vi "Mock Circulation Loop.vi"() -> ()   [LabVIEW 2024]
uses:
  <vilib>/DAQmx/write.llb/DAQmx Write (Analog DBL 1Chan 1Samp).vi
  <vilib>/DAQmx/read.llb/DAQmx Read (Analog 1D DBL NChan 1Samp).vi
  <vilib>/DAQmx/write.llb/DAQmx Write (Digital 1D Bool NChan 1Samp 1Line).vi
  <vilib>/DAQmx/create/channels.llb/DAQmx Create Channel (DO-Digital Output).vi
  <vilib>/DAQmx/miscellaneous.llb/DAQmx Fill In Error Info.vi
  <vilib>/DAQmx/create/channels.llb/DAQmx Create Channel (AI-Voltage-Basic).vi
  <vilib>/DAQmx/create/channels.llb/DAQmx Create Channel (AO-Voltage-Basic).vi
  <vilib>/Utility/file.llb/Write Delimited Spreadsheet (string).vi
  <vilib>/Utility/file.llb/Write Delimited Spreadsheet (DBL).vi
panel:
  in  "Set pressure Hybrid Heart (Bar)":dbl
  in  "Analog output pressure regulator":tag
  out "Actual pressure to Hybrid Heart (Bar)":dbl
  out "Flow sensors":cluster{dbl[], dbl[]}[](graph)
  in  "Seconds per data point":dbl
  out "Pressure sensors":cluster{dbl[], dbl[]}[](graph)
  out "Elapsed time":dbl
  in  "Input port all sensors":tag
  in  "Start/Stop solenoid valves":bool
  in  "Closed time (ms)":dbl
  in  "Open time (ms)":dbl
  in  "STOP":bool
  in  "line grouping":i32(ring)=1 items=["one channel for each line", "one channel for all lines"]
  in  "Port input Solenoid valve":tag
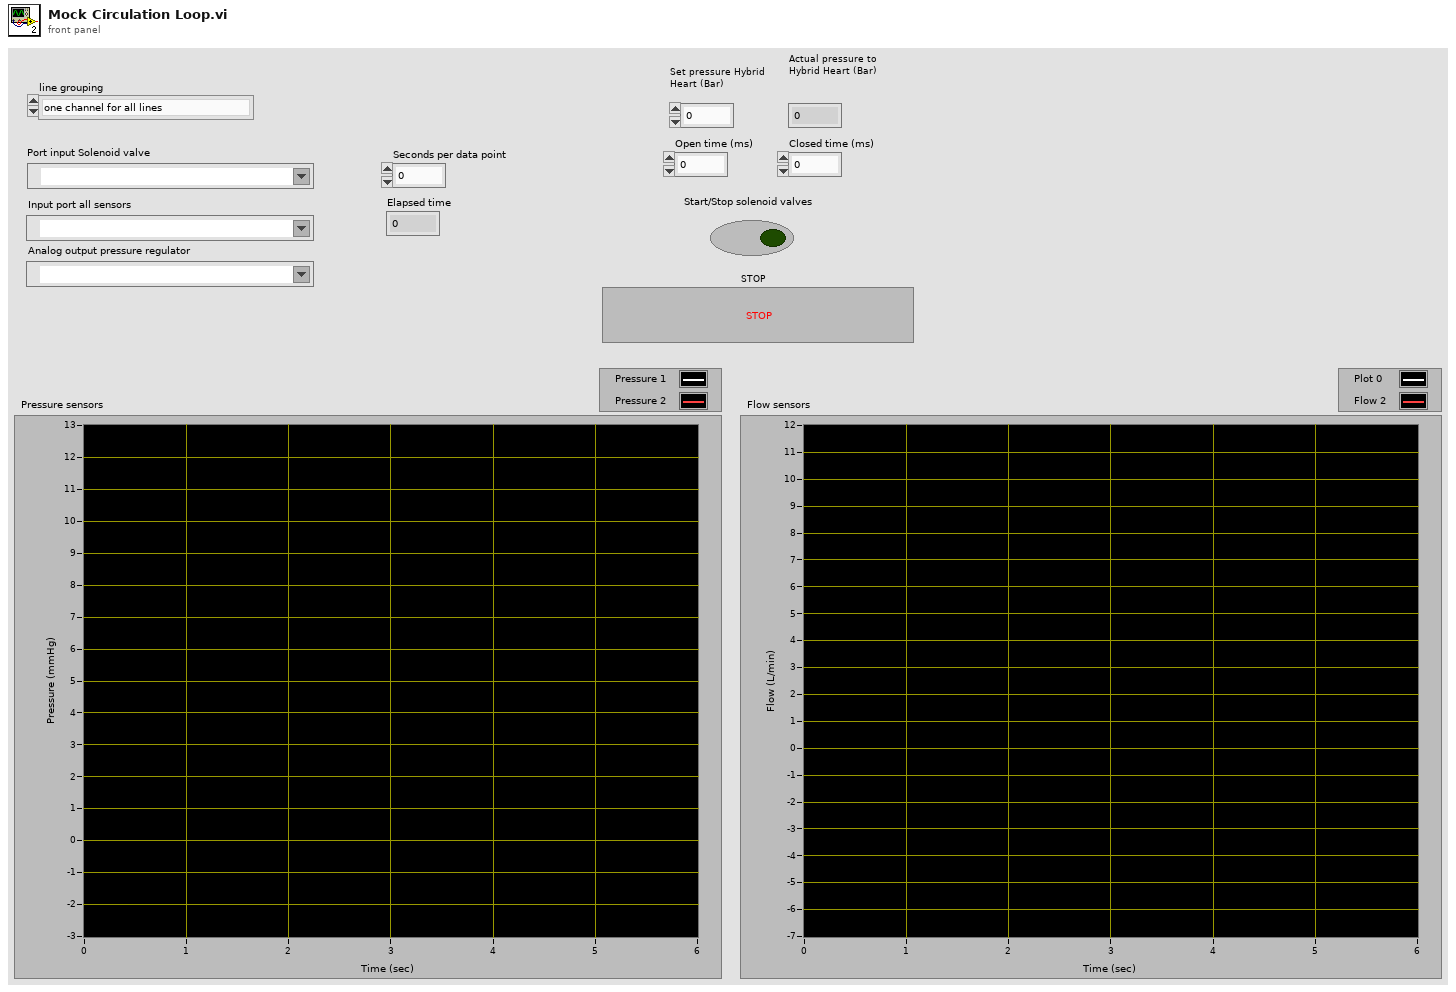
[diagram p1: front panel]
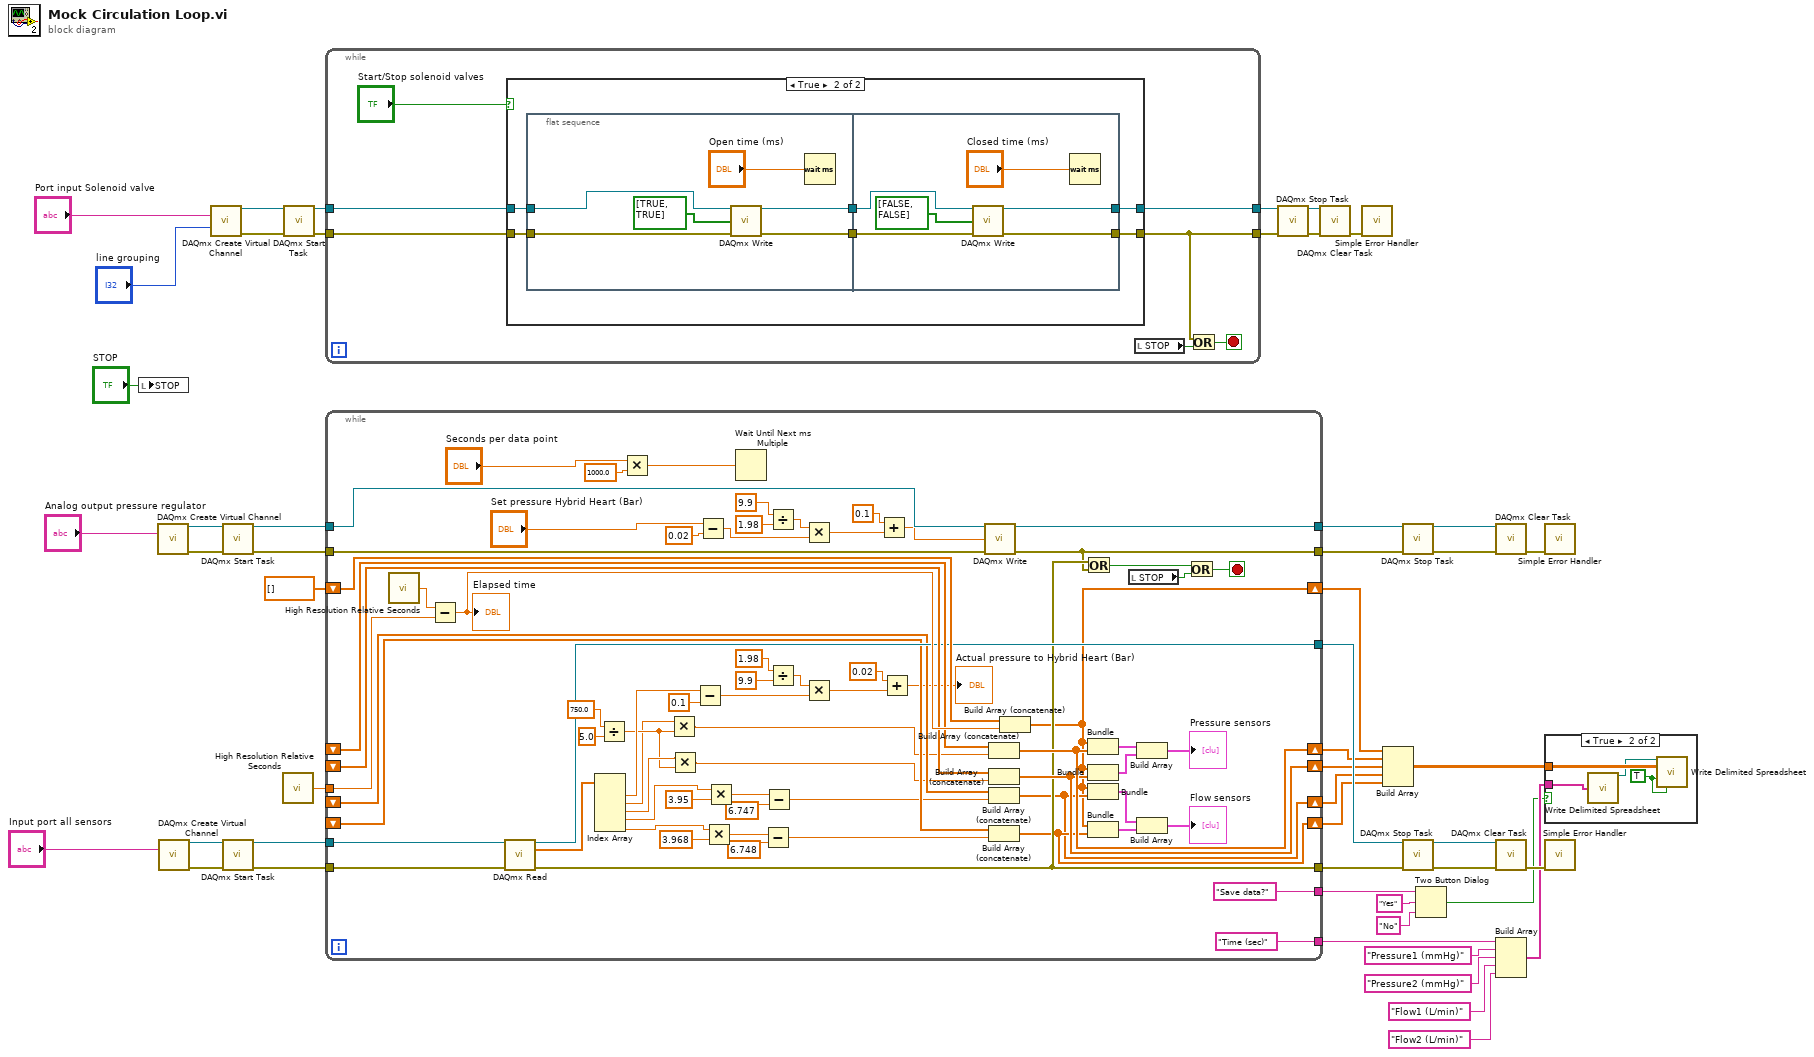
[diagram p0: block diagram]
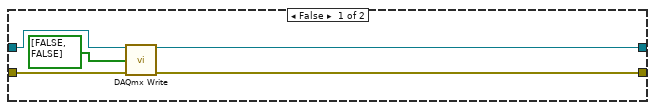
[diagram p3: hidden frame]
diagram:
  n1 = local write "STOP"("STOP") -> ()
  n2 = call-poly <vilib>:"DAQmx Create Virtual Channel.vi"("physical channels"="Analog output pressure regulator") -> ("task out"=w27:refnum<k21>, "error out"=w26:errorcluster)  [unwired: 13 in]
  n3 = call-poly <vilib>:"DAQmx Create Virtual Channel.vi"("physical channels"="Input port all sensors") -> ("task out"=w36:refnum<k21>, "error out"=w35:errorcluster)  [unwired: 13 in]
  n4 = call-poly <vilib>:"DAQmx Create Virtual Channel.vi"("lines"="Port input Solenoid valve", "line grouping"="line grouping") -> ("task out"=w48:refnum<k21>, "error out"=w49:errorcluster)  [unwired: 12 in]
  n5 = call <vilib>:"DAQmx Start Task.vi"("task/channels in"=w27, "error in"=w26) -> ("task out"=w23:refnum<k21>, "error out"=w24:errorcluster)  [unwired: 12 in]
  n6 = call <vilib>:"DAQmx Start Task.vi"("task/channels in"=w36, "error in"=w35) -> ("task out"=w34:refnum<k21>, "error out"=w33:errorcluster)  [unwired: 12 in]
  n7 = call <vilib>:"High Resolution Relative Seconds.vi"() -> ("relative seconds"=w38:dbl)
  n8 = call <vilib>:"DAQmx Start Task.vi"("task/channels in"=w48, "error in"=w49) -> ("task out"=w46:refnum<k21>, "error out"=w45:errorcluster)  [unwired: 12 in]
  n9 = while {
    tunnel: w46 -> [w56]
    tunnel: w45 -> [w55]
    tunnel: [w52] -> w43
    tunnel: [w54] -> w42
    stop <- w53 stop-if-true
    n10 = case shown="True" "Start/Stop solenoid valves" {
      tunnel: w56 -> [w62 w66]
      tunnel: w55 -> [w61 w65]
      tunnel: [w59 w64] -> w52
      tunnel: [w58 w63] -> w54
      frame False {
        n11 = call-poly <vilib>:"DAQmx Write.vi"("task/channels in"=w62, "data"=bool[] [FALSE, FALSE], "error in"=w61) -> ("task out"=w58:refnum<k21>, "error out"=w59:errorcluster)  [unwired: 10 in, 1 out]
      }
      frame True {
        n12 = flat-sequence {
          tunnel: w66 -> [w74]
          tunnel: w65 -> [w73]
          tunnel: [w71] -> w68
          tunnel: [w70] -> w67
          tunnel: w68 -> [w79]
          tunnel: w67 -> [w78]
          tunnel: [w77] -> w63
          tunnel: [w76] -> w64
          frame #0 {
            n13 = call-poly <vilib>:"DAQmx Write.vi"("task/channels in"=w74, "data"=bool[] [TRUE, TRUE], "error in"=w73) -> ("task out"=w71:refnum<k21>, "error out"=w70:errorcluster)  [unwired: 10 in, 1 out]
            n14 = Wait (ms)(milliseconds to wait="Open time (ms)") -> ()  [unwired: 1 out]
          }
          frame #1 {
            n15 = call-poly <vilib>:"DAQmx Write.vi"("task/channels in"=w79, "data"=bool[] [FALSE, FALSE], "error in"=w78) -> ("task out"=w77:refnum<k21>, "error out"=w76:errorcluster)  [unwired: 10 in, 1 out]
            n16 = Wait (ms)(milliseconds to wait="Closed time (ms)") -> ()  [unwired: 1 out]
          }
        }
      }
    }
    n17 = local read "STOP"() -> (w51:bool)
    n18 = Or(x=w52, y=w51) -> (x .or. y?=w53:bool)
  }
  n19 = while {
    tunnel: w34 -> [w151]
    tunnel: w33 -> [w150]
    tunnel: w38 -> [w145]
    shift-right: [w128] -> w17
    shift-left: dbl[] [] -> [w143]
    shift-right: [w139] -> w16
    shift-left: _ -> [w141]
    shift-right: [w138] -> w15
    shift-left: _ -> [w140]
    tunnel: [w134] -> w32
    tunnel: [w133] -> w31
    shift-right: [w129] -> w14
    shift-left: _ -> [w132]
    shift-right: [w130] -> w13
    shift-left: _ -> [w131]
    tunnel: w24 -> [w124]
    tunnel: w23 -> [w123]
    tunnel: [w121] -> w19
    tunnel: [w122] -> w18
    tunnel: ["Time (sec)"] -> w6
    tunnel: ["Save data?" ("message")] -> w2
    stop <- w100 stop-if-true
    n20 = call <vilib>:"High Resolution Relative Seconds.vi"() -> ("relative seconds"=w146:dbl)
    n21 = Subtract(x=w146, y=w145) -> (x-y=w144:dbl)
    "Elapsed time" <- w144
    n22 = call-poly <vilib>:"DAQmx Read.vi"("task/channels in"=w151, "error in"=w150) -> ("task out"=w134:refnum<k21>, "data"=w142:dbl[], "error out"=w133:errorcluster)  [unwired: 11 in]
    n23 = Index Array(array=w142) -> (element #1=w120:dbl, element #2=w81:dbl, element #3=w87:dbl, element #4=w83:dbl, element #5=w82:dbl)  [unwired: 5 in]
    n24 = Divide(x=750.0, y=5.0) -> (x/y=w84:dbl)
    n25 = Multiply(x="Seconds per data point", y=1000.0) -> (x*y=w149:dbl)
    n26 = Multiply(x=w81, y=w84) -> (x*y=w89:dbl)
    n27 = Multiply(x=w87, y=w84) -> (x*y=w88:dbl)
    n28 = Subtract(x=w120, y=0.1) -> (x-y=w119:dbl)
    n29 = Subtract(x="Set pressure Hybrid Heart (Bar)", y=0.02) -> (x-y=w111:dbl)
    n30 = Multiply(x=w82, y=3.968) -> (x*y=w93:dbl)
    n31 = Multiply(x=w83, y=3.95) -> (x*y=w97:dbl)
    n32 = Wait Until Next ms Multiple(millisecond multiple=w149) -> ()  [unwired: 1 out]
    n33 = Subtract(x=w93, y=6.748) -> (x-y=w94:dbl)
    n34 = Subtract(x=w97, y=6.747) -> (x-y=w98:dbl)
    n35 = Divide(x=9.9, y=1.98) -> (x/y=w109:dbl)
    n36 = Divide(x=1.98, y=9.9) -> (x/y=w116:dbl)
    n37 = Multiply(x=w109, y=w111) -> (x*y=w108:dbl)
    n38 = Multiply(x=w116, y=w119) -> (x*y=w115:dbl)
    n39 = Add(x=0.1, y=w108) -> (x+y=w105:dbl)
    n40 = Add(x=0.02, y=w115) -> (x+y=→"Actual pressure to Hybrid Heart (Bar)":dbl)
    n41 = call-poly <vilib>:"DAQmx Write.vi"("task/channels in"=w123, "data"=w105, "error in"=w124) -> ("task out"=w122:refnum<k21>, "error out"=w121:errorcluster)  [unwired: 10 in, 1 out]
    n42 = Build Array (concatenate)(w141, w89) -> (w139:dbl[])
    n43 = Build Array (concatenate)(w140, w88) -> (w138:dbl[])
    n44 = Build Array (concatenate)(w132, w98) -> (w129:dbl[])
    n45 = Build Array (concatenate)(w131, w94) -> (w130:dbl[])
    n46 = Build Array (concatenate)(w143, w144) -> (w128:dbl[])
    n47 = Or(x=w133, y=w121) -> (x .or. y?=w101:bool)
    n48 = Bundle(w128, w139) -> (w137:cluster{dbl[], dbl[]})  [unwired: 1 in]
    n49 = Bundle(w128, w138) -> (w136:cluster{dbl[], dbl[]})  [unwired: 1 in]
    n50 = Bundle(w128, w129) -> (w127:cluster{dbl[], dbl[]})  [unwired: 1 in]
    n51 = Bundle(w128, w130) -> (w126:cluster{dbl[], dbl[]})  [unwired: 1 in]
    n52 = local read "STOP"() -> (w99:bool)
    n53 = Build Array(w137, w136) -> (→"Pressure sensors":cluster{dbl[], dbl[]}[])
    n54 = Build Array(w127, w126) -> (→"Flow sensors":cluster{dbl[], dbl[]}[])
    n55 = Or(x=w101, y=w99) -> (x .or. y?=w100:bool)
  }
  n56 = call <vilib>:"DAQmx Stop Task.vi"("task/channels in"=w42, "error in"=w43) -> ("task out"=w41:refnum<k21>, "error out"=w40:errorcluster)  [unwired: 12 in]
  n57 = call <vilib>:"DAQmx Clear Task.vi"("task in"=w41, "error in"=w40) -> ("error out"=w44:errorcluster)  [unwired: 13 in]
  n58 = call <vilib>:"Simple Error Handler.vi"("error in (no error)"=w44) -> ()  [unwired: 4 in, 5 out]
  n59 = Build Array(w17, w16, w15, w14, w13) -> (w12:dbl[][])
  n60 = call <vilib>:"DAQmx Stop Task.vi"("task/channels in"=w18, "error in"=w19) -> ("task out"=w21:refnum<k21>, "error out"=w22:errorcluster)  [unwired: 12 in]
  n61 = call <vilib>:"DAQmx Stop Task.vi"("task/channels in"=w32, "error in"=w31) -> ("task out"=w29:refnum<k21>, "error out"=w30:errorcluster)  [unwired: 12 in]
  n62 = Two Button Dialog(message=w2, 1:"No" ("F button name (\"Cancel\")"), 2:"Yes" ("T button name (\"OK\")")) -> (T button?=w5:bool)
  n63 = call <vilib>:"DAQmx Clear Task.vi"("task in"=w21, "error in"=w22) -> ("error out"=w20:errorcluster)  [unwired: 13 in]
  n64 = call <vilib>:"DAQmx Clear Task.vi"("task in"=w29, "error in"=w30) -> ("error out"=w28:errorcluster)  [unwired: 13 in]
  n65 = Build Array(w6, "Pressure1 (mmHg)", "Pressure2 (mmHg)", "Flow1 (L/min)", "Flow2 (L/min)") -> (w7:string[])
  n66 = call <vilib>:"Simple Error Handler.vi"("error in (no error)"=w20) -> ()  [unwired: 4 in, 5 out]
  n67 = case shown="True" w5 {
    tunnel: w12 -> [_ w155]
    tunnel: w7 -> [_ w154]
    frame False {
    }
    frame True {
      w152 = TRUE ("transpose? (no:F)")
      n68 = call-poly <vilib>:"Write Delimited Spreadsheet.vi"("1D data"=w154) -> ("new file path (Not A Path if cancelled)"=w153:path)  [unwired: 13 in, 1 out]
      n69 = call-poly <vilib>:"Write Delimited Spreadsheet.vi"("file path (dialog if empty)"=w153, "2D data"=w155, "append to file? (new file:F)"=w152, "transpose? (no:F)"=w152) -> ()  [unwired: 10 in, 2 out]
    }
  }
  n70 = call <vilib>:"Simple Error Handler.vi"("error in (no error)"=w28) -> ()  [unwired: 4 in, 5 out]
